vi "Init.vi"(8 "error in (no error)":errorcluster, 10 "Address":string, 11 "HamaCam in":refnum<class "HamaCam.lvclass">) -> (0 "error out":errorcluster, 3 "HamaCam out":refnum<class "HamaCam.lvclass">)   [LabVIEW 2023, in "HamaCam.lvlib" / "HamaCam.lvclass"]
uses:
  HamaCam.lvclass
  HamaCam.lvclass/HamaCam.ctl
  Interfaces/InitDeinitInterface/InitDeinitComm Messages/InitDone Msg/InitDone Msg.lvclass
  <vilib>/ActorFramework/Actor/Actor.lvclass
  UIs/InterferometryUI/InterferometryUI/instrumentType.ctl
  Applications/National Instruments/LabVIEW 2023 64-bit/vi.lib/ActorFramework/Actor/Actor.lvclass
  Users/alexandrosspiliotis/Documents/LV_DAQ_Project/ConcreteClasses/ConcreteInstrumentClasses/CameraClasses/Hama_LV/HamaCam/HamaCam/HamaCam.lvclass
  Users/alexandrosspiliotis/Documents/LV_DAQ_Project/Interfaces/AbstractInstrumentClasses/Cameras_LV/CameraInterface/CameraInterface.lvclass
  Users/alexandrosspiliotis/Documents/LV_DAQ_Project/Interfaces/InitDeinitInterface/InitDeinit/InitDeinit.lvclass
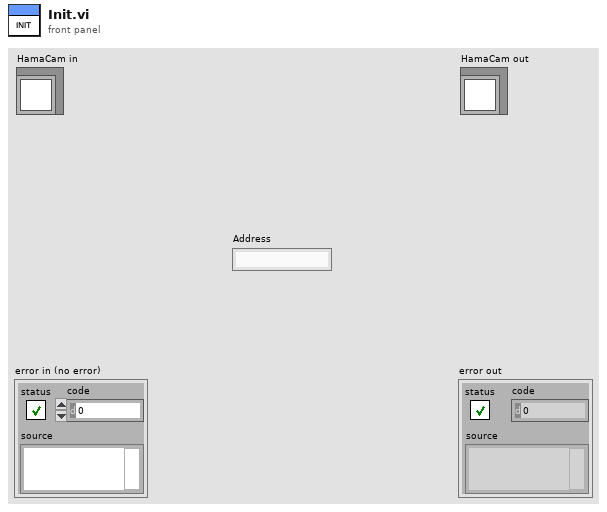
[diagram p1: front panel]
types:
  T1 = typedef "instrumentType.ctl" = enum16{"Spectrometer", "Camera", "Stepper"}
  T2 = cluster{"Model":string, "Camera ID":string, "Firmware":string}
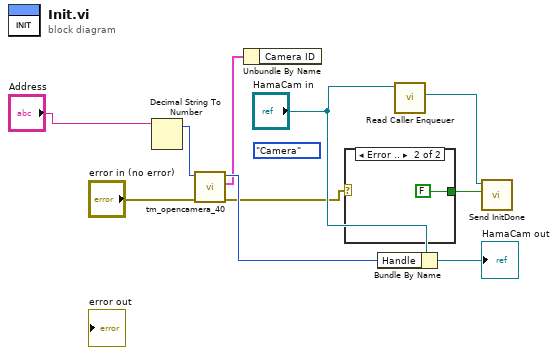
[diagram p0: block diagram]
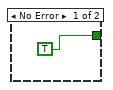
[diagram p2: hidden frame]
diagram:
  (unwired) instrumentType."Camera" ("instrument type")
  n1 = Decimal String To Number(string="Address") -> (offset past number=w10:i32)  [unwired: 2 in, 1 out]
  n2 = call "tm_opencamera_40.vi"("error in (no error)"="error in (no error)", "Camera Index"=w10) -> ("error out"=w2:errorcluster, "Camera Details"=w6:T2, "Handle out"=w8:u32)  [unwired: 7 in]
  n3 = Unbundle By Name(w6) -> ()  [unwired: 1 out]
  n4 = case shown="Error .." w2 {
    tunnel: [TRUE FALSE] -> w1
    frame No Error {
    }
    frame Error {
    }
  }
  n5 = Bundle By Name(cluster="HamaCam in", "Handle"=w8) -> (→"HamaCam out":refnum<class "HamaCam.lvclass">)
  n6 = call <vilib>:"Read Caller Enqueuer.vi"("Actor"="HamaCam in") -> ("Caller Enqueuer"=w5:refnum<class "Message Enqueuer.lvclass">)  [unwired: 10 in]
  n7 = call "Send InitDone.vi"("Initialized"=w1, "Message Enqueuer"=w5) -> ()  [unwired: 8 in, 2 out]
